vi "configure.vi"(8 "error in (no error)":errorcluster, 11 "StimulatorDL090727DAQmx in":refnum<class "StimulatorDL090727Writer.lvclass">) -> (0 "error out":errorcluster, 3 "StimulatorDL090727DAQmx out":refnum<class "StimulatorDL090727Writer.lvclass">)   [LabVIEW 2010, in "StimulatorDL090727Writer.lvclass"]
doc: "The dynamic dispatch version of this VI loads and displays the configuration file associated with the plug-in object. The user modify and save the configuration data."
uses:
  StimulatorDL090727Writer.lvclass
  common/xcontrols/XComponentSpecification/XComponentSpecification/XComponentSpecification.xctl
  StimulatorDL090727Writer.lvclass/StimulatorDL090727Writer.ctl
  SignalWriter/GenericSignalWriter/GenericSignalWriter/GenericSignalWriter.lvclass
  Clock/GenericClock/GenericClock/GenericClock.lvclass
  common/classes/GenericComponent/GenericComponent/GenericComponent.lvclass
panel:
  out "configuration":string
  in  "save button":bool
  in  "cancel button":bool
  in  "Tab Control":T1(tab)
  in  "output writer spec":T2(xcontrol)
  in  "sampling rate":dbl[unit]
  in  "clock spec":T2(xcontrol)
  # "Configure Stimulator090727DAQmx"
  # "This component generates a stimulator pattern via a National Instruments DAQ card."
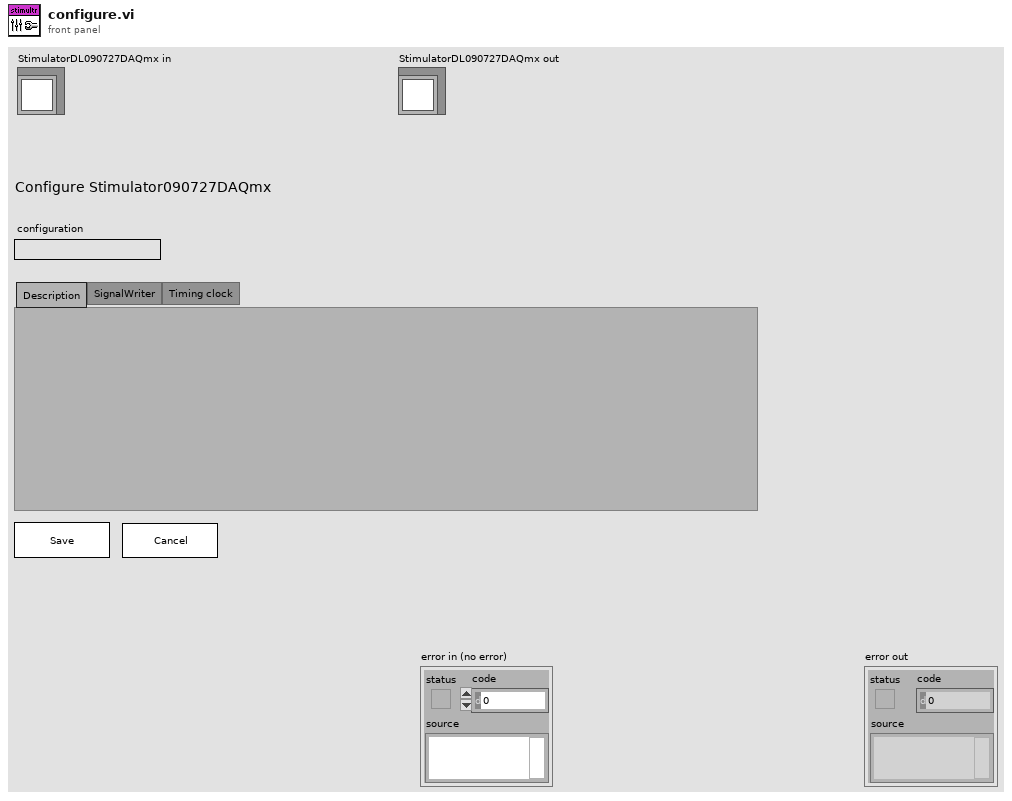
[diagram p1: front panel]
types:
  T1 = enum32{"Description", "SignalWriter", "Timing clock"}
  T2 = cluster{"class path":string, "configuration":string, "label":string, "settings name":string}
  T3 = typedef "plugin_specification.ctl" = cluster{"class path":string, "configuration":string, "label":string, "settings name":string}
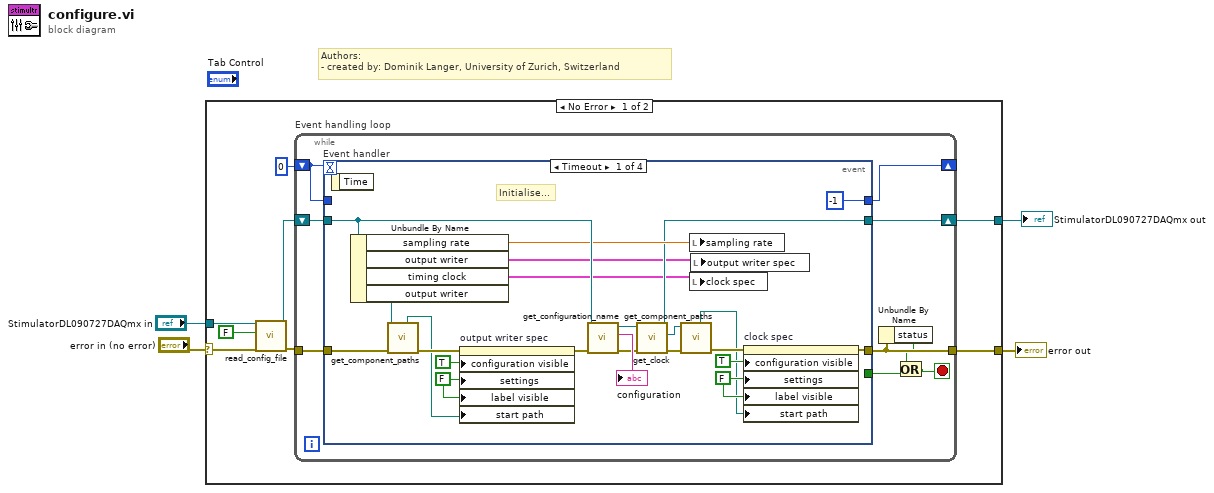
[diagram p0: block diagram]
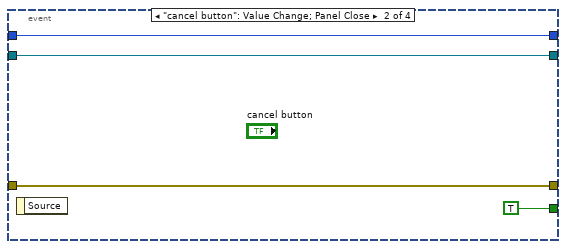
[diagram p2: hidden frame]
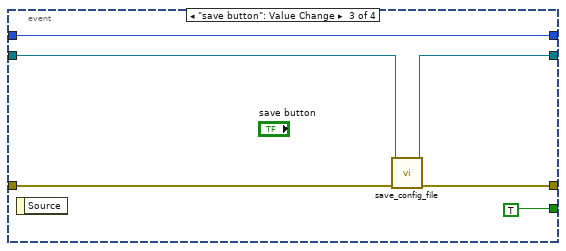
[diagram p3: hidden frame]
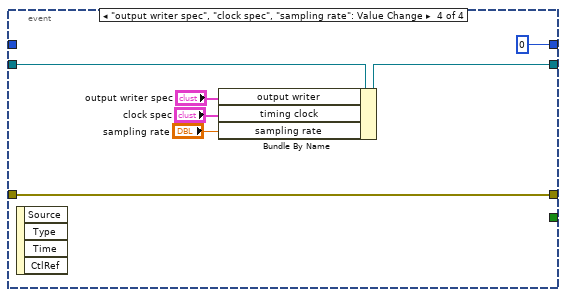
[diagram p4: hidden frame]
diagram:
  # "Authors: \n- created by: Dominik Langer, University of Zurich, Switzerland"
  n1 = case shown="No Error" "error in (no error)" {
    selector: "error in (no error)" -> [w8 w63]
    tunnel: [w12 w63] -> w3
    tunnel: "StimulatorDL090727DAQmx in" -> [w6 w62]
    tunnel: [w10 w62] -> w1
    frame No Error {
      n2 = call-dynamic "read_config_file.vi"("error in (no error)"=w8, "force load?"=FALSE, "GenericPlugin in"=w6) -> ("error out"=w7:errorcluster, "GenericPlugin out"=w5:refnum<class "StimulatorDL090727Writer.lvclass">)  [unwired: 7 in]
      n3 = while "Event handling loop" {
        shift-right: [w19] -> _
        shift-left: 0 -> [w20]
        shift-right: [w17] -> w10
        shift-left: w5 -> [w18]
        tunnel: w7 -> [w21]
        tunnel: [w16] -> w12
        stop <- w13 stop-if-true
        n4 = event "Event handler" shown="[0] Timeout" {
          selector: _ -> [_ _ _ _]
          dyn-events: _ -> [_ _ _ _]
          timeout: w20 -> [_ _ _ _]
          tunnel: w21 -> [w40 w48 w52 w57]
          tunnel: [w26 w48 w50 w57] -> w16
          tunnel: w20 -> [_ w47 w54 _]
          tunnel: [-1 w47 w54 0] -> w19
          tunnel: [_ TRUE TRUE _] -> w15
          tunnel: w18 -> [w43 w45 w49 w61]
          tunnel: [w35 w45 w51 w60] -> w17
          event Timeout {
            w28 = FALSE ("configuration visible")
            w29 = FALSE ("configuration visible")
            # "Initialise..."
            n5 = event-data() -> ()  [unwired: 2 out]
            n6 = Unbundle By Name(w43) -> ("sampling rate"=w41:dbl[unit], "output writer"=w23:T3, "timing clock"=w22:T3, "output writer"=w39:refnum<class "GenericSignalWriter.lvclass">)
            n7 = call-dynamic "get_component_paths.vi"("error in (no error)"=w40, "GenericComponent in"=w39) -> ("error out"=w33:errorcluster, "component type directory"=w32:path)  [unwired: 4 in, 4 out]
            n8 = property on="output writer spec" class="XComponentSpecification (strict"(error in=w33, "configuration visible"=TRUE, "settings"=w29, "label visible"=w29, "start path"=w32) -> (error out=w31:errorcluster)  [unwired: 1 in, 1 out]
            n9 = call "get_configuration_name.vi"("error in (no error)"=w31, "GenericPlugin.lvclass in"=w43) -> ("error out"=w38:errorcluster, "configuration name"=→"configuration":string, "GenericPlugin.lvclass out"=w36:refnum<class "StimulatorDL090727Writer.lvclass">)  [unwired: 7 in]
            n10 = call-dynamic "get_clock.vi"("error in (no error)"=w38, "Stimulator090724Scaffold in"=w36) -> ("error out"=w37:errorcluster, "clock"=w34:refnum<class "GenericClock.lvclass">, "Stimulator090724Scaffold out"=w35:refnum<class "StimulatorDL090727Writer.lvclass">)  [unwired: 7 in]
            n11 = call-dynamic "get_component_paths.vi"("error in (no error)"=w37, "GenericComponent in"=w34) -> ("error out"=w25:errorcluster, "component type directory"=w24:path)  [unwired: 4 in, 4 out]
            n12 = local write "sampling rate"(w41) -> ()
            n13 = local write "clock spec"(w22) -> ()
            n14 = local write "output writer spec"(w23) -> ()
            n15 = property on="clock spec" class="XComponentSpecification (strict"(error in=w25, "configuration visible"=TRUE, "settings"=w28, "label visible"=w28, "start path"=w24) -> (error out=w26:errorcluster)  [unwired: 1 in, 1 out]
          }
          event "cancel button": Value Change; Panel Close {
            n16 = event-data() -> ()  [unwired: 2 out]
          }
          event "save button": Value Change {
            n17 = event-data() -> ()  [unwired: 2 out]
            n18 = call-dynamic "save_config_file.vi"("error in (no error)"=w52, "GenericPlugin in"=w49) -> ("error out"=w50:errorcluster, "GenericPlugin out"=w51:refnum<class "StimulatorDL090727Writer.lvclass">)  [unwired: 8 in]
          }
          event "output writer spec", "clock spec", "sampling rate": Value Change {
            n19 = event-data() -> ()  [unwired: 5 out]
            n20 = Bundle By Name(cluster=w61, "output writer"="output writer spec", "timing clock"="clock spec", "sampling rate"="sampling rate") -> (w60:refnum<class "StimulatorDL090727Writer.lvclass">)
          }
        }
        n21 = Unbundle By Name(w16) -> ("status"=w14:bool)
        n22 = Or(x=w14, y=w15) -> (x .or. y?=w13:bool)
      }
    }
    frame Error {
    }
  }
  "error out" <- w3
  "StimulatorDL090727DAQmx out" <- w1
